vi "Numerical Representations Limits.vi"() -> ()   [LabVIEW 2020]
uses:
  6e073f0a-beec-4b33-8ea9-aca74cba6d32.vi
panel:
  out "maximum value for type":u16
  out "minimum value for type":u16
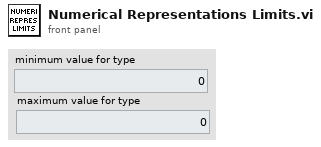
[diagram p1: front panel]
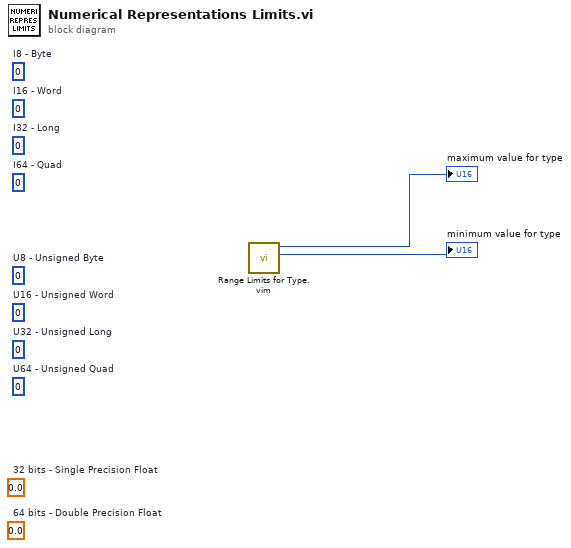
[diagram p0: block diagram]
diagram:
  (unwired) 0.0  # 64 bits - Double Precision Float
  (unwired) sgl 0.0  # 32 bits - Single Precision Float
  (unwired) i64 0  # U64 - Unsigned Quad
  (unwired) 0  # U32 - Unsigned Long
  (unwired) i16 0  # U16 - Unsigned Word
  (unwired) i8 0  # U8 - Unsigned Byte
  (unwired) i64 0  # I64 - Quad
  (unwired) 0  # I32 - Long
  (unwired) i16 0  # I16 - Word
  (unwired) i8 0  # I8 - Byte
  n1 = call "Range Limits for Type.vim"() -> ("minimum value for type"=→"minimum value for type":u16, "maximum value for type"=→"maximum value for type":u16)  [unwired: 10 in]
